vi "Draw Pendulum.vi"(10 "Target":T2={"Position"=0.2, "Invert"=TRUE} {"Position" min=-0.5 max=0.5 step=0.1 format="%.2g"}, 11 "States In":T1 format="%.4f") -> (2 "Picture":picture)   [LabVIEW 2018]
uses:
  Target.ctl
  States.ctl
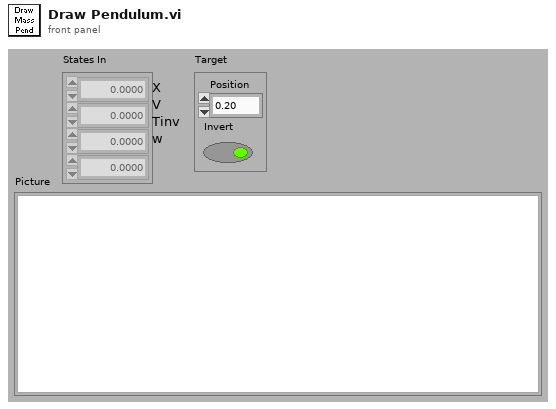
[diagram p1: front panel]
types:
  T1 = typedef "States.ctl" = dbl[]
  T2 = typedef "Target.ctl" = cluster{"Position":dbl, "Invert":bool}
  T3 = cluster{"Width":u16, "Style":enum32{"Solid", "Dash", "Dot", "DashDot", "DashDotDot"}}
  T4 = cluster{"Width":i16, "Style":enum32{"Solid", "Dash", "Dot", "DashDot", "DashDotDot"}}
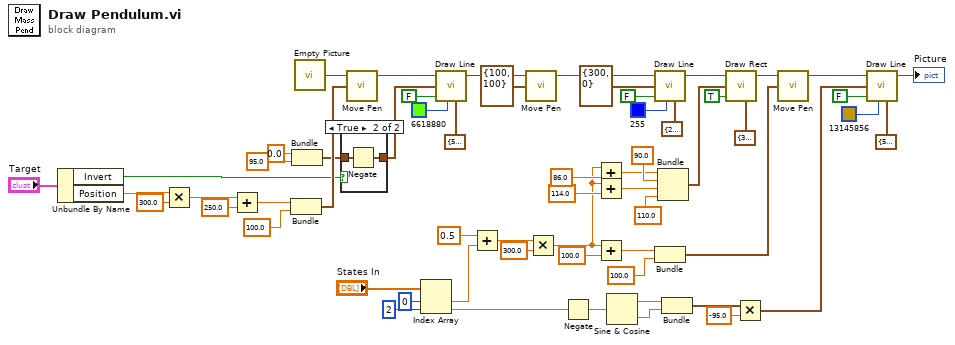
[diagram p0: block diagram]
diagram:
  n1 = Unbundle By Name("Target") -> ("Invert"=w19:bool, "Position"=w26:dbl)
  n2 = Multiply(x=w26, y=300.0) -> (x*y=w31:dbl)
  n3 = Add(x=w31, y=250.0) -> (x+y=w29:dbl)
  n4 = Bundle(w29, "y"=100.0) -> (w23:cluster{dbl, "y":dbl})  [unwired: 1 out]
  n5 = Bundle("y"=0.0, "y"=95.0) -> (w21:cluster{"y":dbl, "y":dbl})  [unwired: 1 out]
  n6 = call "Empty Picture"() -> ("empty picture"=w12:picture)
  n7 = case shown="True" w19 {
    tunnel: w21 -> [w61 w63]
    tunnel: [w61 w62] -> w20
    frame False {
    }
    frame True {
      n8 = Negate(x=w63) -> (-x=w62:cluster{"y":dbl, "y":dbl})
    }
  }
  n9 = call <vilib>:"Move Pen.vi"("new position"=w23, "picture"=w12) -> ("new picture"=w24:picture)  [unwired: 1 in, 2 out]
  n10 = Index Array(array="States In", index #1=0 ("index"), index #2=2 ("index")) -> (element #1=w7:dbl, element #2=w6:dbl)
  n11 = call <vilib>:"Draw Line.vi"("picture"=w24, "end point"=w20, "absolute coordinates?(T)"=FALSE, "color(black)"=u32 6618880, "pen"=T3 {"Width"=5, "Style"=enum."Solid"}) -> ("new picture"=w11:picture)  [unwired: 4 out]
  n12 = Add(x=0.5, y=w7) -> (x+y=w33:dbl)
  n13 = call <vilib>:"Move Pen.vi"("new position"=cluster{"x":i16, "y":i16} {"x"=100, "y"=100}, "picture"=w11) -> ("new picture"=w37:picture)  [unwired: 1 in, 2 out]
  n14 = Multiply(x=w33, y=300.0) -> (x*y=w42:dbl)
  n15 = Negate(x=w6) -> (-x=w35:dbl)
  n16 = Add(x=w42, y=86.0 ("y 3")) -> (x+y=w41:dbl)
  n17 = Add(x=w42, y=114.0 ("y 4")) -> (x+y=w53:dbl)
  n18 = Add(x=w42, y=100.0) -> (x+y=w48:dbl)
  n19 = Sine & Cosine(0:w35) -> (1:w45:dbl, 2:w44:dbl)
  n20 = call <vilib>:"Draw Line.vi"("picture"=w37, "end point"=cluster{"x":i16, "y":i16} {"x"=300, "y"=0}, "absolute coordinates?(T)"=FALSE, "color(black)"=u32 255, "pen"=T3 {"Width"=2, "Style"=enum."Solid"}) -> ("new picture"=w13:picture)  [unwired: 4 out]
  n21 = Bundle(w48, "y"=100.0) -> (w46:cluster{dbl, "y":dbl})  [unwired: 1 out]
  n22 = Bundle(w41, "y"=90.0, w53, "y 2"=110.0) -> (w50:cluster{dbl, "y":dbl, dbl, "y 2":dbl})  [unwired: 1 out]
  n23 = Bundle(w45, w44) -> (w57:cluster{dbl, dbl})  [unwired: 1 out]
  n24 = call <vilib>:"Draw Rect.vi"("picture"=w13, "rect"=w50, "fill?(F)"=TRUE, "pen"=T4 {"Width"=3, "Style"=enum."Solid"}) -> ("new picture"=w60:picture)  [unwired: 1 in, 4 out]
  n25 = Multiply(x=w57, y=-95.0) -> (x*y=w56:cluster{dbl, dbl})
  n26 = call <vilib>:"Move Pen.vi"("new position"=w46, "picture"=w60) -> ("new picture"=w59:picture)  [unwired: 1 in, 2 out]
  n27 = call <vilib>:"Draw Line.vi"("picture"=w59, "end point"=w56, "absolute coordinates?(T)"=FALSE, "color(black)"=u32 13145856, "pen"=T3 {"Width"=5, "Style"=enum."Solid"}) -> ("new picture"=→"Picture":picture)  [unwired: 4 out]
